vi "map inputs.vi"(8 "Error In":errorcluster, 10 "CD state in":T1[](array[typedef])) -> (0 "Error Out":errorcluster, 2 "CD state out":T1[](array[typedef]))   [LabVIEW 2014, in "UEGO Sim Engine.lvlib"]
uses:
  UEGO Sim Engine.lvlib
  UEGO CD state.ctl
  Shared/UEGO fpga inputs.ctl
  Shared/UEGO fpga outputs.ctl
  Shared/VS input channels.ctl
  Shared/VS output channels.ctl
  Shared/UEGO Sim Shared.lvlib
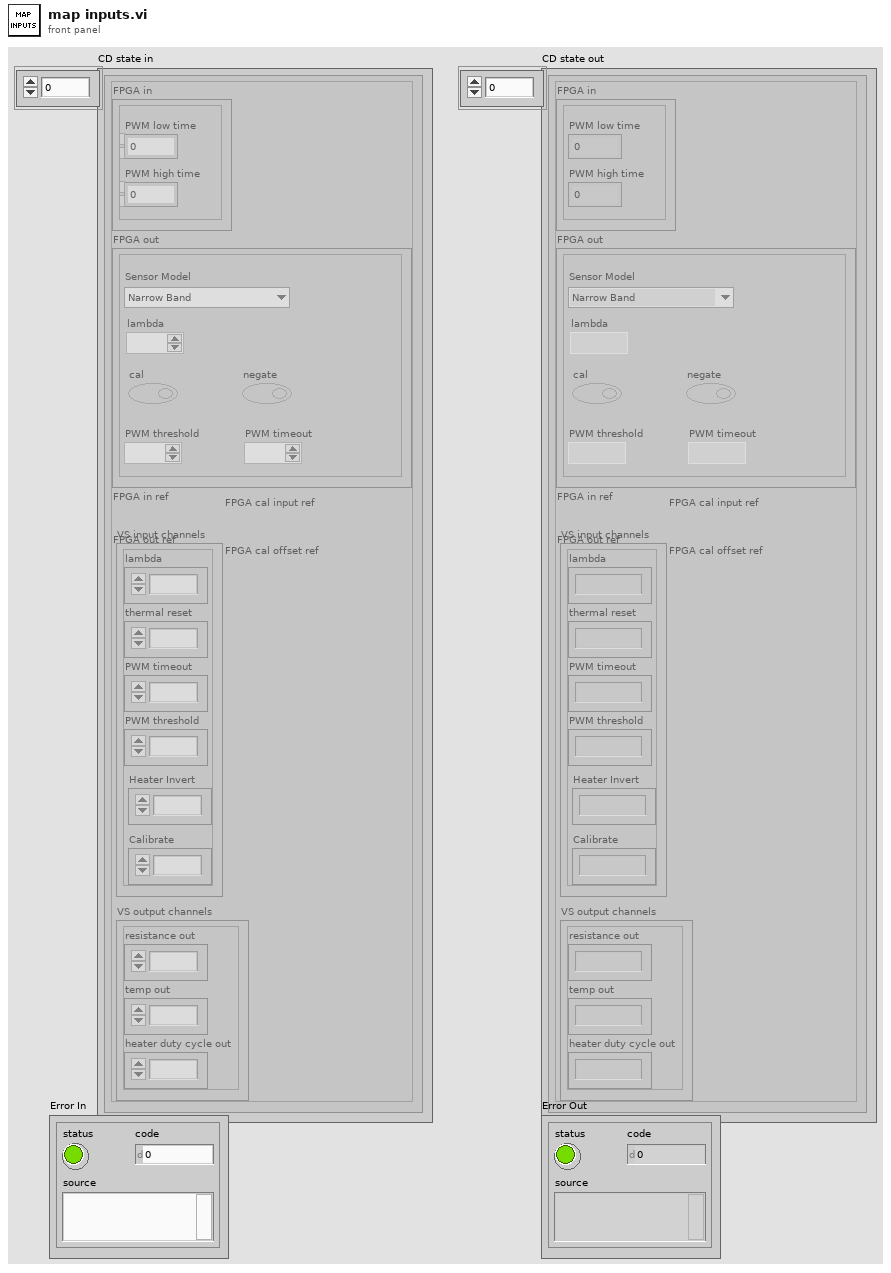
[diagram p1: front panel]
types:
  T1 = typedef "UEGO Sim Engine.lvlib/UEGO CD state.ctl" = cluster{"FPGA in":T2, "FPGA out":T3, "FPGA in ref":refnum<k20>, "FPGA out ref":refnum<k20>, "VS input channels":T5, "VS output channels":T6, "FPGA cal input ref":refnum<k20>, "FPGA cal offset ref":refnum<k20>}
  T2 = typedef "UEGO Sim Shared.lvlib/UEGO fpga inputs.ctl" = cluster{"PWM low time":u32, "PWM high time":u32}
  T3 = typedef "UEGO Sim Shared.lvlib/UEGO fpga outputs.ctl" = cluster{"Sensor Model":T4, "lambda":fxp<+,12,3>, "cal":bool, "negate":bool, "PWM threshold":i16, "PWM timeout":u32}
  T4 = typedef "UEGO Sim Shared.lvlib/sensor models" = enum16{"Narrow Band", "Bosch 4.2", "Bosch 4.9"}
  T5 = typedef "UEGO Sim Shared.lvlib/VS input channels.ctl" = cluster{"lambda":dbl, "thermal reset":dbl, "PWM timeout":dbl, "PWM threshold":dbl, "Heater Invert":dbl, "Calibrate":dbl}
  T6 = typedef "UEGO Sim Shared.lvlib/VS output channels.ctl" = cluster{"resistance out":dbl, "temp out":dbl, "heater duty cycle out":dbl}
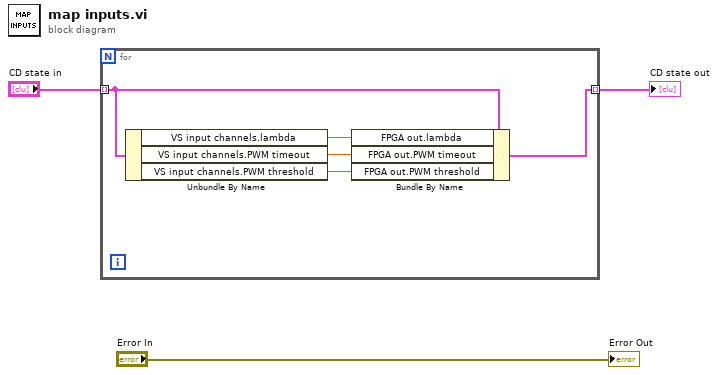
[diagram p0: block diagram]
diagram:
  n1 = for {
    tunnel: "CD state in" -> [w7] mode=indexing
    tunnel: [w6] -> w2 mode=indexing
    n2 = Unbundle By Name(w7) -> ("VS input channels.lambda"=w8:dbl, "VS input channels.PWM timeout"=w5:dbl, "VS input channels.PWM threshold"=w4:dbl)
    n3 = Bundle By Name(cluster=w7, "FPGA out.lambda"=w8, "FPGA out.PWM timeout"=w5, "FPGA out.PWM threshold"=w4) -> (w6:T1)
  }
  "CD state out" <- w2
  "Error Out" <- "Error In"
